vi "Tetra_BOUNCE_Close.vi"() -> (0 "error out":errorcluster={"status"=FALSE, "code"=1073676418, "source"="VISA Close in Tetra_RX-PROD_Close.vi"}, 2 "Status":string="Setting up Power Supplies...ERROR!...\rDone !!!\n...Shut Off RF\rDONE!!!")   [LabVIEW 2018]
uses:
  <vilib>/Utility/error.llb/DialogType.ctl
  Initialize References/Station References Global.vi
  Tetra_Globals.vi
  Instruments/Keysight N6700/Agilent N6700 Series/Agilent N6700 Series.lvlib
  Infrastructure/Test Parameter Globals_1.0.0.vi
panel:
  in  "close serial(t)":bool=TRUE
  in  "Close Oven(t)":bool=TRUE
  out "Text":refnum<vi>
  in  "Close Power Supply (T)":bool=TRUE
  in  "error in (no error)":errorcluster
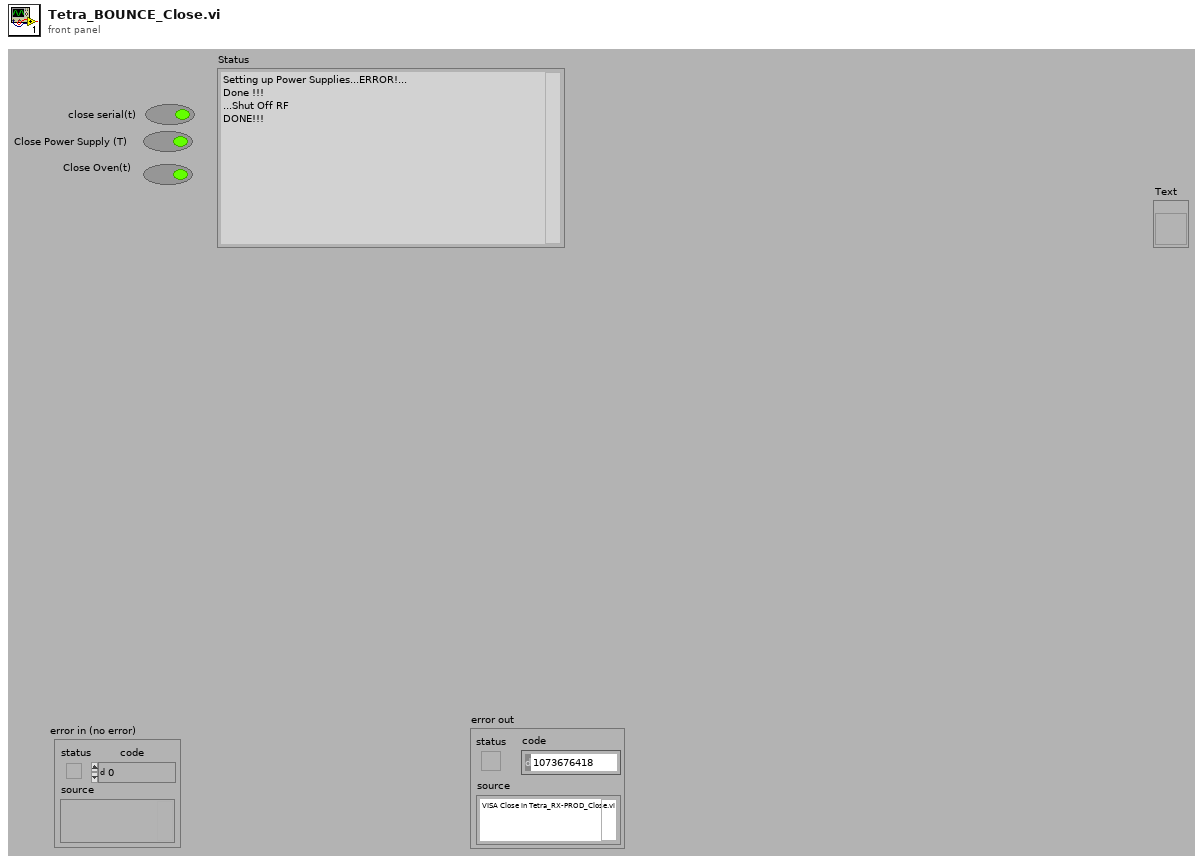
[diagram p1: front panel]
types:
  T1 = typedef "DialogType.ctl" = u16
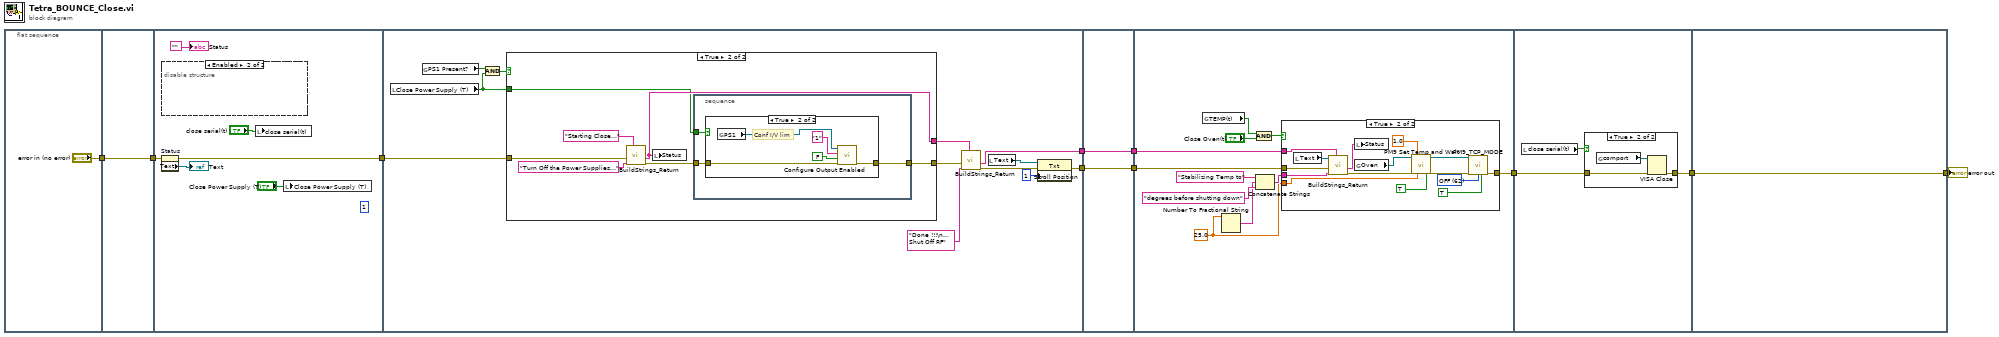
[diagram p0: block diagram]
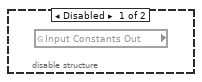
[diagram p2: hidden frame]
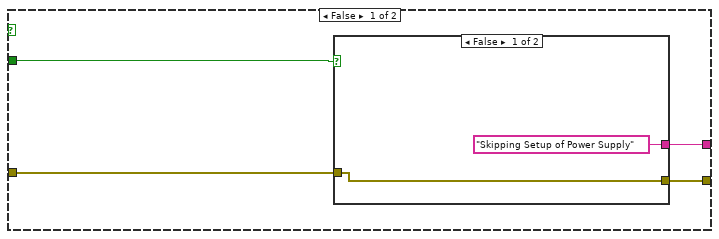
[diagram p3: hidden frame]
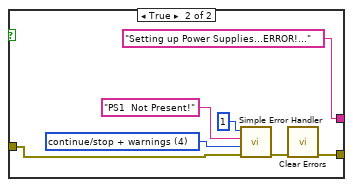
[diagram p4: hidden frame]
diagram:
  n1 = flat-sequence {
    tunnel: ["error in (no error)"] -> w4
    tunnel: w4 -> [w12]
    tunnel: [w12] -> w3
    tunnel: [w15] -> w9
    tunnel: w3 -> [w14]
    tunnel: [w30] -> w5
    tunnel: w9 -> [w26]
    tunnel: [w21] -> w2
    tunnel: [w60] -> w6
    tunnel: [w61] -> w8
    tunnel: w5 -> [w61]
    tunnel: w2 -> [w60]
    tunnel: w8 -> [w69]
    tunnel: [w64] -> w7
    tunnel: w6 -> [w68]
    tunnel: w7 -> [w91]
    tunnel: [w90] -> w1
    tunnel: [w96] -> w10
    tunnel: w1 -> [w96]
    frame #0 {
    }
    frame #1 {
    }
    frame #2 {
      (unwired) u32 1 ("Text.Scroll Position")
      n2 = disable-structure shown="Enabled" {
        frame Disabled {
          n3 = global read "Test Parameter Globals_1.0.0.vi" "Input Constants Out"() -> ()  [unwired: 1 out]
        }
        frame Enabled {
        }
      }
      n4 = property on="Status" class="Str"(error in=w14) -> (error out=w15:errorcluster, "Text"=→"Text":refnum<vi>)  [unwired: 1 in, 1 out]
      n5 = local write "close serial(t)"("close serial(t)") -> ()
      n6 = local write "Close Power Supply (T)"("Close Power Supply (T)") -> ()
      "Status" <- ""
    }
    frame #3 {
      n7 = local read "Close Power Supply (T)"() -> (w22:bool)
      n8 = global read "Station References Global.vi" "PS1 Present?"() -> (w25:bool)
      n9 = And(x=w25, y=w22) -> (x .and. y?=w23:bool)
      n10 = case shown="True" w23 {
        tunnel: [w34 w46] -> w19
        tunnel: w26 -> [w33 w48]
        tunnel: [w32 w45] -> w20
        tunnel: w22 -> [w31 w44]
        frame False {
          n11 = case shown="False" w31 {
            tunnel: [w36 w39] -> w34
            tunnel: w33 -> [w36 w38]
            tunnel: ["Skipping Setup of Power Supply" "Setting up Power Supplies...ERROR!..."] -> w32
            frame False {
            }
            frame True {
              w41 = T1 4 items=["no dialog", "OK message", "continue or stop message", "OK message + warnings", "continue/stop + warnings"] ("type of dialog (OK msg:1)")
              n12 = call <vilib>:"Simple Error Handler.vi"("error code (no error:0)"=1, "error source (\" \")"="PS1  Not Present!" ("error source (\" \")"), "type of dialog (OK msg:1)"=w41, "error in (no error)"=w38) -> ("error out"=w40:errorcluster)  [unwired: 1 in, 4 out]
              n13 = call <vilib>:"Clear Errors.vi"("error in (no error)"=w40) -> ("error out"=w39:errorcluster)  [unwired: 5 in, 1 out]
            }
          }
        }
        frame True {
          n14 = call "BuildStrings_Return.vi"("Input String"="Starting Close...", "New String"="Turn Off the Power Supplies...", "error in (no error)"=w48) -> ("error out"=w47:errorcluster, "concatenated string"=w45:string)  [unwired: 6 in, 1 out]
          n15 = local write "Status"(w45) -> ()
          n16 = stacked-sequence {
            tunnel: w47 -> [w53]
            tunnel: [w52] -> w46
            tunnel: w44 -> [w51]
            frame #0 {
              n17 = case shown="True" w51 {
                tunnel: [w54 w57] -> w52
                tunnel: w53 -> [w54 w56]
                frame False {
                }
                frame True {
                  # "Conf I/V lim"
                  n18 = global read "Station References Global.vi" "PS1"() -> (w55:refnum<visa-resource-name>)
                  n19 = call "Configure Output Enabled.vi"("error in (no error)"=w56, "Enable Output (False)"=FALSE, "Channel Name (1)"="1", "VISA resource name"=w55) -> ("error out"=w57:errorcluster)  [unwired: 6 in, 1 out]
                }
              }
            }
          }
        }
      }
      n20 = call "BuildStrings_Return.vi"("Input String"=w20, "New String"="Done !!!\n...Shut Off RF", "error in (no error)"=w19) -> ("error out"=w27:errorcluster, "concatenated string"=w21:string)  [unwired: 6 in, 1 out]
      n21 = local read "Text"() -> (w29:refnum<vi>)
      n22 = property class="Txt"(reference=w29, error in=w27, "Scroll Position"=u32 1) -> (error out=w30:errorcluster)  [unwired: 1 out]
    }
    frame #4 {
    }
    frame #5 {
      w62 = 25.0 ("Set Point")
      n23 = global read "Tetra_Globals.vi" "TEMP(t)"() -> (w66:bool)
      n24 = Number To Fractional String(number=w62) -> (F-format string=w63:string)  [unwired: 3 in]
      n25 = And(x=w66, y="Close Oven(t)") -> (x .and. y?=w65:bool)
      n26 = Concatenate Strings("Stabilizing Temp to" ("New String"), w63, "degrees before shutting down" ("string")) -> (w67:string)
      n27 = case shown="True" w65 {
        tunnel: w69 -> [w73 w85]
        tunnel: w68 -> [_ w87]
        tunnel: w67 -> [_ w86]
        tunnel: [w73 w78] -> w64
        tunnel: w62 -> [_ w75]
        frame False {
        }
        frame True {
          w80 = u16 62 items=["READ ONLY"=0, "AUTO"=10, "OFF"=62, "MAN"=54] ("MODE")
          n28 = local read "Text"() -> (w76:refnum<vi>)
          n29 = call "BuildStrings_Return.vi"("Input String"=w87, "New String"=w86, "error in (no error)"=w85, "reference"=w76) -> ("error out"=w84:errorcluster, "concatenated string"=w82:string)  [unwired: 5 in, 1 out]
          n30 = local write "Status"(w82) -> ()
          n31 = global read "Station References Global.vi" "Oven"() -> (w88:refnum<visa-resource-name>)
          n32 = call "PM9 Set Temp and Wait.vi"("VISA"=w88, "Error In"=w84, "Accuracy +/-"=1.0, "Set Point"=w75, "close session(t)"=TRUE) -> ("visa"=w77:refnum<visa-resource-name>, "error out"=w81:errorcluster)  [unwired: 11 in, 2 out]
          n33 = call "PM9_TCP_MODE.vi"("VISA"=w77, "error in (no error)"=w81, "MODE"=w80, "Close tcp(t)"=TRUE) -> ("error out"=w78:errorcluster)  [unwired: 8 in, 3 out]
        }
      }
    }
    frame #6 {
      n34 = local read "close serial(t)"() -> (w89:bool)
      n35 = case shown="True" w89 {
        tunnel: w91 -> [w92 w94]
        tunnel: [w92 w93] -> w90
        frame False {
        }
        frame True {
          n36 = global read "Tetra_Globals.vi" "comport"() -> (w95:refnum<visa-resource-name>)
          n37 = VISA Close(VISA resource name=w95, error in (no error)=w94) -> (error out=w93:errorcluster)
        }
      }
    }
    frame #7 {
    }
  }
  "error out" <- w10
